vi "Create Plugin Groups.vi"(8 "error in (no error)":errorcluster, 9 "String":string, 10 "dsf refnum in":refnum<class "Configuration Session.lvclass">, 11 "Section Ptr":T1 format="%.0x") -> (0 "error out":errorcluster)   [LabVIEW 2017, in "DSF System Explorer.lvlib"]
uses:
  DSF System Explorer.lvlib
  <vilib>/NI Veristand/Custom Device API/Custom Device Item Ref.ctl
  DSF Core.lvlibp/Classes/Configuration/Configuration Session.lvclass
  DSF Core.lvlibp/Classes/Configuration/Read Plugin Group IDs.vi
  Shared/Group Page GUID.vi
  <vilib>/NI Veristand/Custom Device API/Set Item Property (String).vi
  DSF Core.lvlibp/Classes/Configuration/Read Group.vi
  <vilib>/NI Veristand/Custom Device API/Custom Device API.lvlib
  Shared/DSF Shared.lvlib
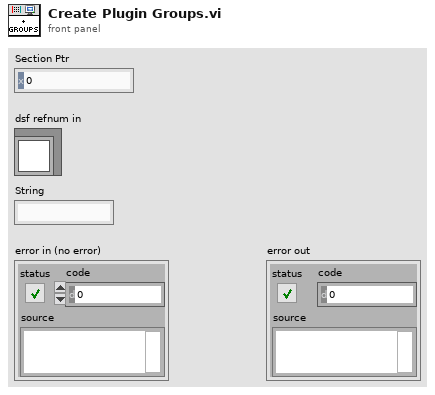
[diagram p1: front panel]
types:
  T1 = typedef "Custom Device API.lvlib/Custom Device Item Ref.ctl" = u64
  T2 = typedef "DSF System Explorer.lvlib/shared data ref.ctl" = refnum<data-value>
  T3 = typedef "DSF Core.lvlibp/DSF Group Info.ctl" = cluster{"direction":T4, "timing":T5, "transfer ids":string[], "settings id":string, "thread":i32, "timeout behavior":T6}
  T4 = typedef "DSF Core.lvlibp/DSF Direction.ctl" = enum8{"Tx", "Rx"}
  T5 = typedef "DSF Core.lvlibp/DSF Timing Info.ctl" = cluster{"priority":u64, "decimation":u64, "offset":u64}
  T6 = typedef "DSF Core.lvlibp/DSF Timeout Behavior.ctl" = enum8{"Increment Late Count", "Throw Error"}
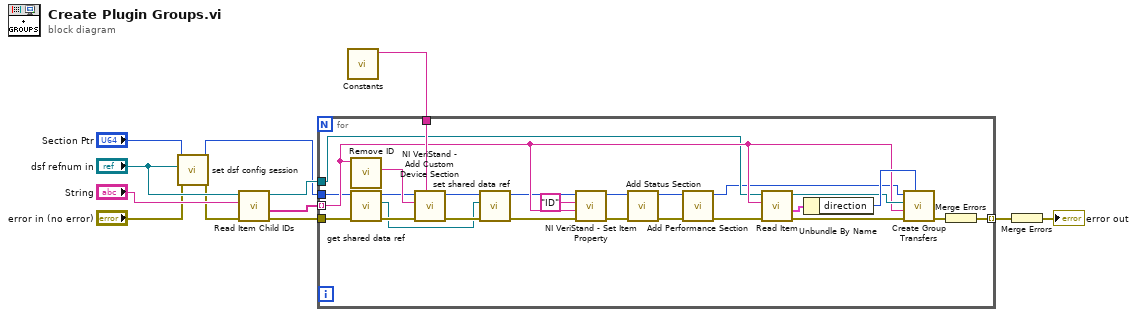
[diagram p0: block diagram]
diagram:
  n1 = call "set dsf config session.vi"("error in (no error)"="error in (no error)", "Configuration Session"="dsf refnum in", "Item Ref in"="Section Ptr") -> ("error out"=w1:errorcluster, "Item Ref out"=w3:T1)  [unwired: 7 in]
  n2 = call-poly "Read Item Child IDs.vi"("error in (no error)"=w1, "Plugin ID"="String", "Configuration Session"="dsf refnum in") -> ("error out"=w9:errorcluster, "Group IDs"=w8:string[], "Configuration Session out"=w7:refnum<class "Configuration Session.lvclass">)  [unwired: 5 in, 1 out]
  n3 = call-poly "Constants.vi"() -> ("Group GUID"=w6:string)  [unwired: 11 in]
  n4 = for {
    tunnel: w8 -> [w29] mode=indexing
    tunnel: w3 -> [w27]
    tunnel: w9 -> [w26]
    tunnel: [w38] -> w12 mode=indexing
    tunnel: w7 -> [w28]
    tunnel: w6 -> [w31]
    n5 = call "Remove ID.vi"("id string"=w29) -> ("name"=w32:string)  [unwired: 8 in, 2 out]
    n6 = call "get shared data ref.vi"("error in (no error)"=w26, "Item Ref in"=w27) -> ("error out"=w25:errorcluster, "shared data ref"=w19:T2, "Item Ref out"=w24:T1)  [unwired: 7 in]
    n7 = call <vilib>:"NI VeriStand - Add Custom Device Section.vi"("GUID (Default Section)"=w31, "error in (no error)"=w25, "Section Name"=w32, "Parent Ref in"=w24) -> ("error out"=w23:errorcluster, "Section Ptr"=w22:T1)  [unwired: 4 in, 2 out]
    n8 = call "set shared data ref.vi"("error in (no error)"=w23, "shared data ref"=w19, "Node Ptr"=w22) -> ("error out"=w20:errorcluster, "Item Ref out"=w21:T1)  [unwired: 7 in]
    n9 = call-poly <vilib>:"NI VeriStand - Set Item Property.vi"("error in (no error)"=w20, "Value"=w29, "Property Name"="ID", "Item Ref in"=w21) -> ("error out"=w18:errorcluster, "Item Ref out"=w17:T1)  [unwired: 5 in, 1 out]
    n10 = call "Add Status Section.vi"("error in (no error)"=w18, "Item Ref in"=w17) -> ("error out"=w16:errorcluster, "Item Ref out"=w14:T1)  [unwired: 8 in]
    n11 = call "Add Performance Section.vi"("error in (no error)"=w16, "Item Ref in"=w14) -> ("error out"=w15:errorcluster, "Item Ref out"=w13:T1)  [unwired: 8 in]
    n12 = call-poly "Read Item.vi"("error in (no error)"=w15, "Group ID"=w29, "Configuration Session in"=w28) -> ("error out"=w34:errorcluster, "value"=w33:T3, "Configuration Session out"=w35:refnum<class "Configuration Session.lvclass">)  [unwired: 5 in, 1 out]
    n13 = Unbundle By Name(w33) -> ("direction"=w37:T4)
    n14 = call "Create Group Transfers.vi"("direction"=w37, "error in (no error)"=w34, "Group ID"=w29, "dsf refnum in"=w35, "Section Ptr"=w13) -> ("error out"=w36:errorcluster)  [unwired: 6 in]
    n15 = Merge Errors(w36) -> (w38:errorcluster)
  }
  n16 = Merge Errors(w12) -> (→"error out":errorcluster)
